vi "test-TimeInterpPose-Test1.vi"() -> (3 "All tests passed":bool)   [LabVIEW 2019]
uses:
  <vilib>/Rock Robotics/WPI/ThirdParty/JAS_Junk/TrajLib/POSE2D.ctl
  <vilib>/Rock Robotics/WPI/ThirdParty/JAS_Junk/TrajLib/TRANSLATION2D.ctl
  <vilib>/Rock Robotics/WPI/ThirdParty/JAS_Junk/TrajLib/ROTATION2D.ctl
  <vilib>/Rock Robotics/WPI/ThirdParty/JAS_Junk/TrajLib/Rotation2d_CreateAngle.vi
  <vilib>/Rock Robotics/WPI/ThirdParty/JAS_Junk/TrajLib/Translation2d_Create.vi
  <vilib>/Rock Robotics/WPI/ThirdParty/JAS_Junk/TrajLib/Translation2d_Equals.vi
  <vilib>/Rock Robotics/WPI/ThirdParty/JAS_Junk/TrajLib/Rotation2d_Equals.vi
  <vilib>/Rock Robotics/WPI/ThirdParty/JAS_Junk/TrajLib/TimeInterpPose2d_CleanUp.vi
  <vilib>/Rock Robotics/WPI/ThirdParty/JAS_Junk/TrajLib/Util_CalcDist.vi
  <vilib>/gmath/interp.llb/Search Ordered Table.vi
  <vilib>/Rock Robotics/WPI/ThirdParty/JAS_Junk/TrajLib/Trajectory_Library.lvlib
panel:
  out "out POSE 1.0":T1 {"ROTATION"."SIN" format="%13.4f"; "ROTATION"."COS" format="%13.4f"; "ROTATION"."VALUE" format="%13.4f"; "TRANSLATION"."Y" format="%14.3f"; "TRANSLATION"."X" format="%14.3f"}
  out "OutputPose 0.75":T1={"TRANSLATION"={"X"=0.0, "Y"=0.0}, "ROTATION"={"VALUE"=0.0, "COS"=1.0, "SIN"=0.0}} {"ROTATION"."SIN" format="%13.4f"; "ROTATION"."COS" format="%13.4f"; "ROTATION"."VALUE" format="%13.4f"; "TRANSLATION"."Y" format="%14.3f"; "TRANSLATION"."X" format="%14.3f"}
  out "out POSE  0.0":T1 {"ROTATION"."SIN" format="%13.4f"; "ROTATION"."COS" format="%13.4f"; "ROTATION"."VALUE" format="%13.4f"; "TRANSLATION"."Y" format="%14.3f"; "TRANSLATION"."X" format="%14.3f"}
  out "OutputPose 0.5":T1={"TRANSLATION"={"X"=0.0, "Y"=0.0}, "ROTATION"={"VALUE"=0.0, "COS"=1.0, "SIN"=0.0}} {"ROTATION"."SIN" format="%13.4f"; "ROTATION"."COS" format="%13.4f"; "ROTATION"."VALUE" format="%13.4f"; "TRANSLATION"."Y" format="%14.3f"; "TRANSLATION"."X" format="%14.3f"}
  out "OutputPose 0.25":T1={"TRANSLATION"={"X"=0.0, "Y"=0.0}, "ROTATION"={"VALUE"=0.0, "COS"=1.0, "SIN"=0.0}} {"ROTATION"."SIN" format="%13.4f"; "ROTATION"."COS" format="%13.4f"; "ROTATION"."VALUE" format="%13.4f"; "TRANSLATION"."Y" format="%14.3f"; "TRANSLATION"."X" format="%14.3f"}
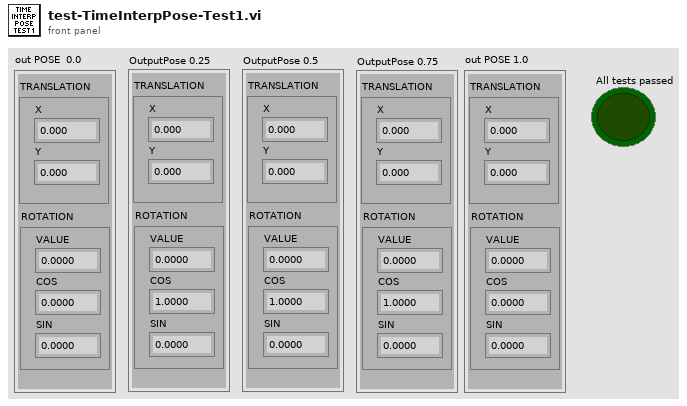
[diagram p1: front panel]
types:
  T1 = typedef "Trajectory_Library.lvlib/POSE2D.ctl" = cluster{"TRANSLATION":T2, "ROTATION":T3}
  T2 = typedef "Trajectory_Library.lvlib/TRANSLATION2D.ctl" = cluster{"X":dbl, "Y":dbl}
  T3 = typedef "Trajectory_Library.lvlib/ROTATION2D.ctl" = cluster{"VALUE":dbl, "COS":dbl, "SIN":dbl}
  T4 = typedef "Trajectory_Library.lvlib/TIME_INTERPOLATABLE_POSE.ctl" = cluster{"TimeStamps":dbl[], "Pose":T1[], "Min_TimeStamp":dbl, "Max_TimeStamp":dbl, "ItemCount":i32, "MaxBufferTime":dbl}
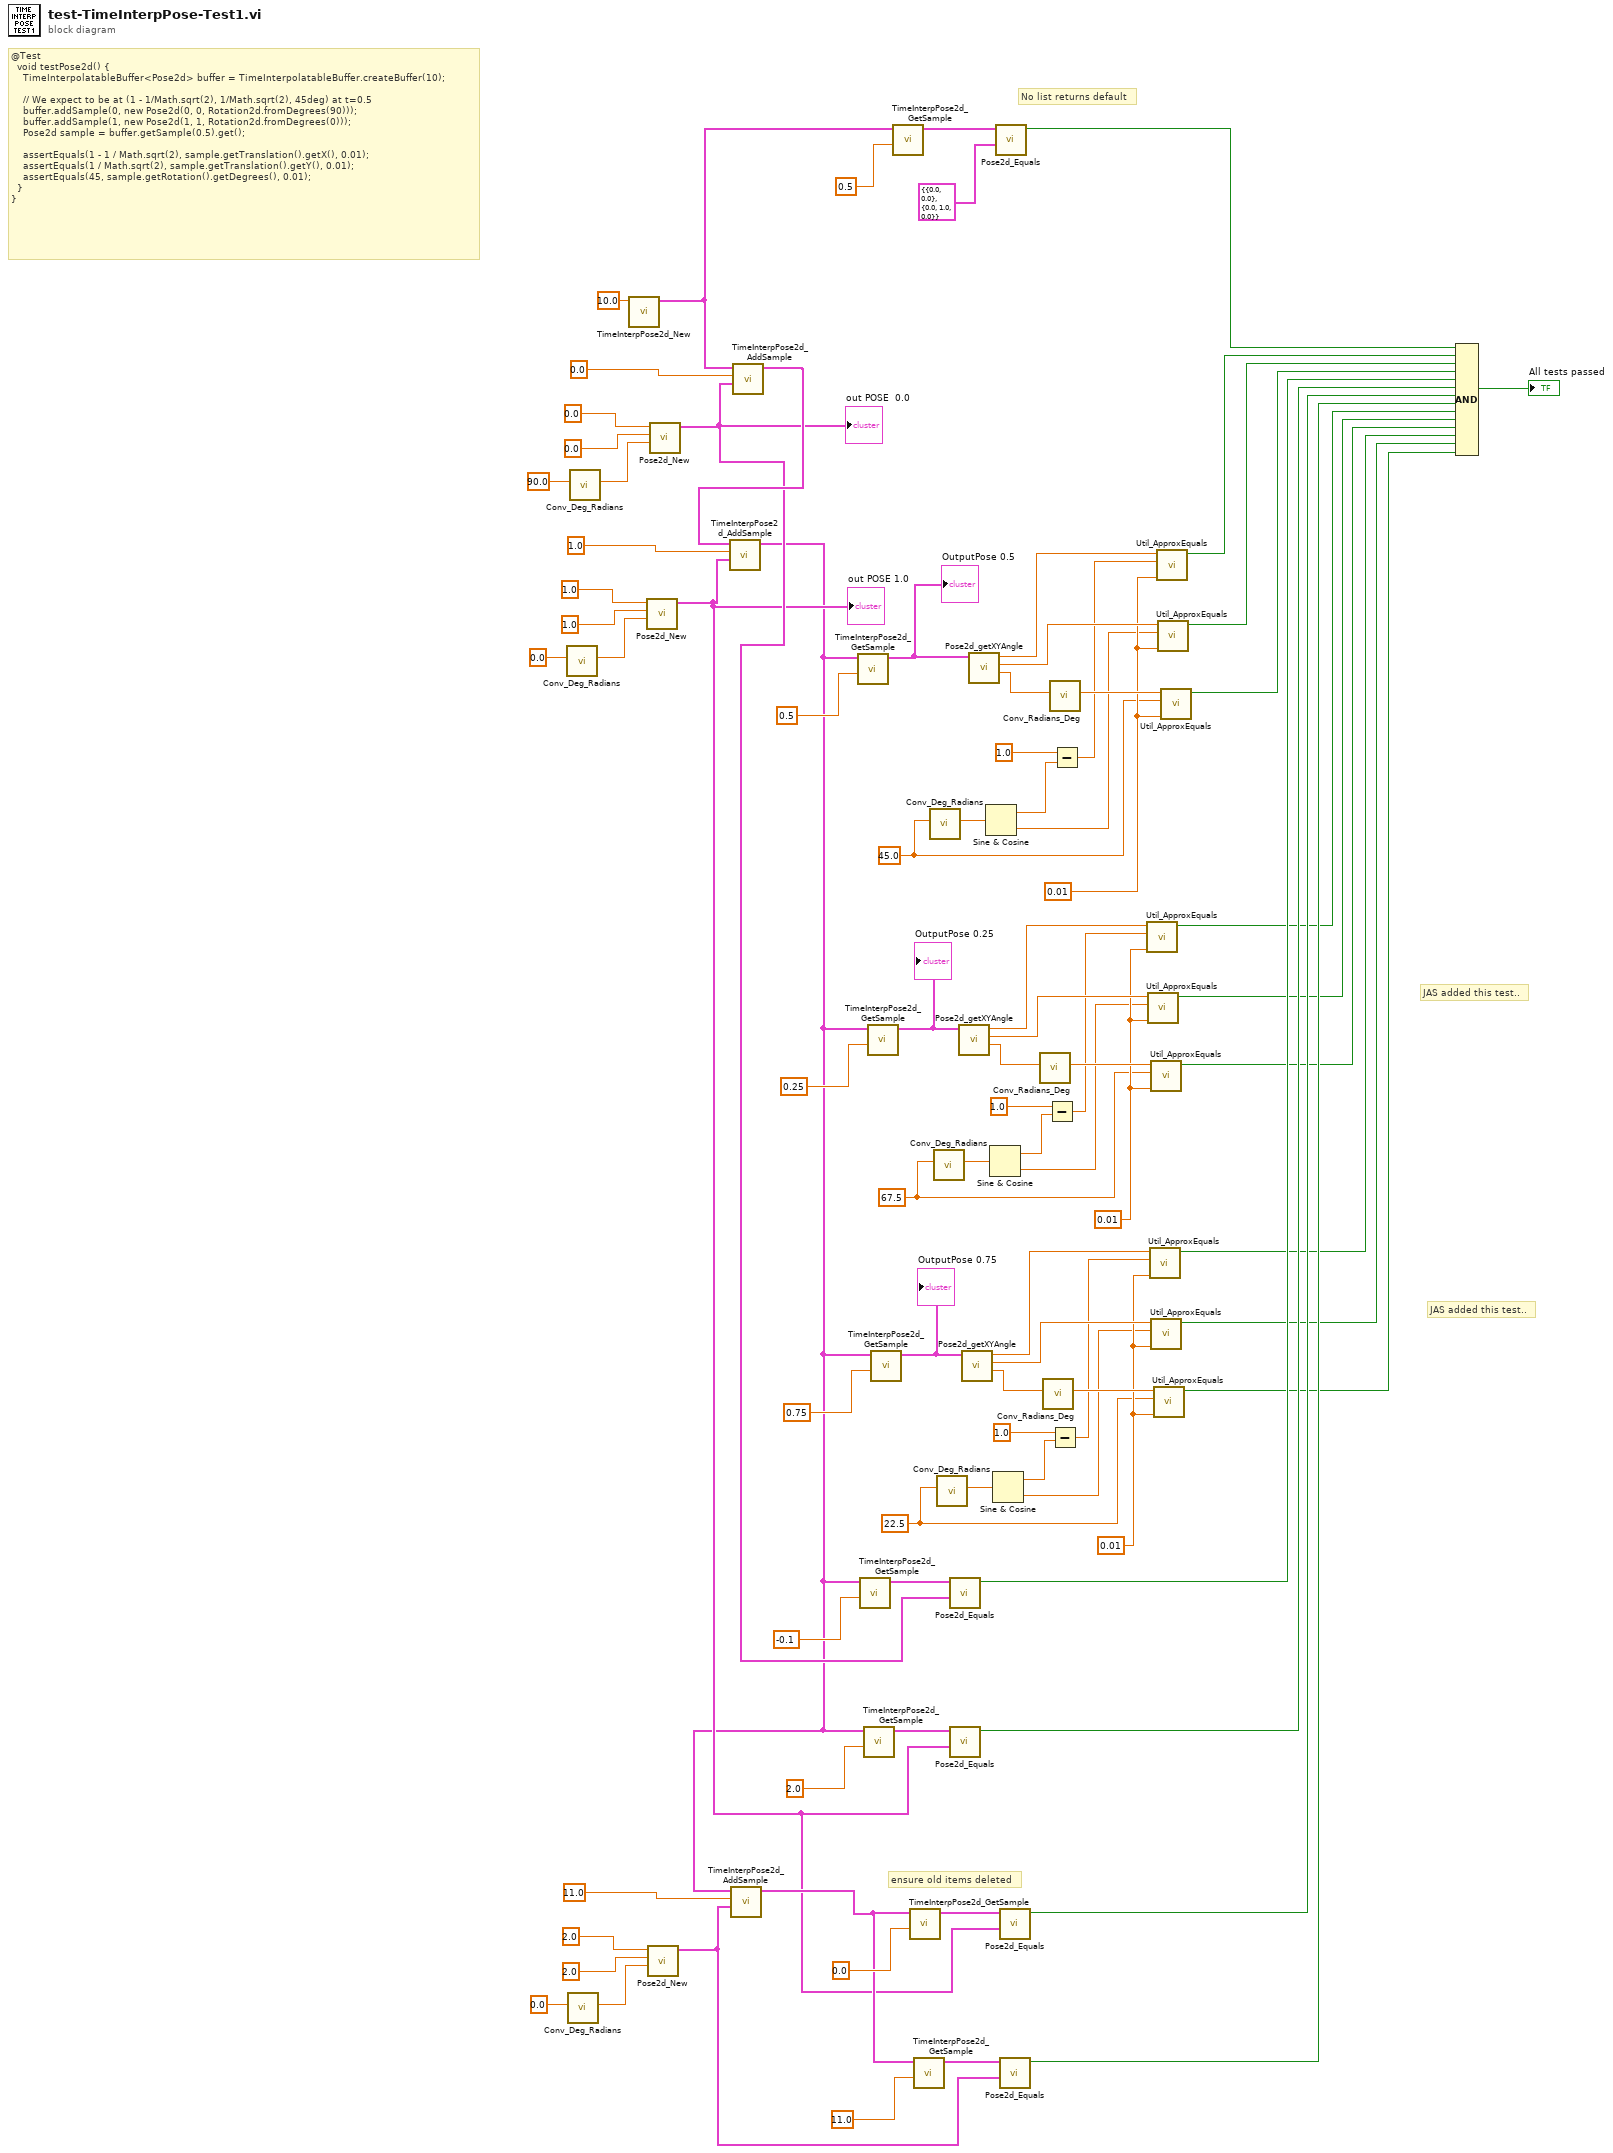
[diagram p0: block diagram]
diagram:
  w9 = 22.5 ("Value 2")
  w11 = 0.01 ("Tolerance")
  w24 = 67.5 ("Value 2")
  w31 = 0.01 ("Tolerance")
  w68 = 0.01 ("Tolerance")
  w27 = 45.0 ("Value 2")
  # "JAS added this test.."
  # "JAS added this test.."
  # "ensure old items deleted"
  # "No list returns default"
  # "@Test\n  void testPose2d() {\n    TimeInterpolatableBuffer<Pose2d> buffer = TimeInterpolatableBuffer.createBuffer(10);\n\n    // We expect to be at (1 - 1/Math.sqrt(2), 1/Math.sqrt(2), 45deg) at t=0.5\n    buffer.addSample(0, new Pose2d(0, 0, Rotation2d.fromDegrees(90)));\n    buffer.addSample(1, new Pose2d(1, 1, Rotation2d.fromDegrees(0)));\n    Pose2d sample = buffer.getSample(0.5).get();\n\n    assertEquals(1 - 1 / Math.sqrt(2), sample.getTranslation().getX(), 0.01);\n    assertEquals(1 / Math.sqrt(2), sample.getTranslation().getY(), 0.01);\n    assertEquals(45, sample.getRotation().getDegrees(), 0.01);\n  }\n}"
  n1 = call <vilib>:"Conv_Deg_Radians.vi"("Degress"=0.0) -> ("Radians"=w79:dbl)  [unwired: 10 in]
  n2 = call <vilib>:"Conv_Deg_Radians.vi"("Degress"=0.0) -> ("Radians"=w49:dbl)  [unwired: 10 in]
  n3 = call <vilib>:"Conv_Deg_Radians.vi"("Degress"=90.0) -> ("Radians"=w84:dbl)  [unwired: 10 in]
  n4 = call <vilib>:"TimeInterpPose2d_New.vi"("MaxTime"=10.0) -> ("TimeInterpPose"=w60:T4)  [unwired: 10 in]
  n5 = call <vilib>:"Pose2d_New.vi"("Heading"=w79, "Y"=1.0, "X"=1.0) -> ("out POSe"=w38:T1)  [unwired: 8 in]
  "out POSE 1.0" <- w38
  n6 = call <vilib>:"Pose2d_New.vi"("Heading"=w49, "Y"=2.0, "X"=2.0) -> ("out POSe"=w41:T1)  [unwired: 8 in]
  n7 = call <vilib>:"Pose2d_New.vi"("Heading"=w84, "Y"=0.0, "X"=0.0) -> ("out POSe"=w56:T1)  [unwired: 8 in]
  "out POSE  0.0" <- w56
  n8 = call <vilib>:"TimeInterpPose2d_AddSample.vi"("Pose"=w56, "TimeStamp"=0.0, "in TimeInterpPose"=w60) -> ("out TimeInterpPose"=w63:T4)  [unwired: 7 in, 1 out]
  n9 = call <vilib>:"TimeInterpPose2d_AddSample.vi"("Pose"=w38, "TimeStamp"=1.0, "in TimeInterpPose"=w63) -> ("out TimeInterpPose"=w4:T4)  [unwired: 7 in, 1 out]
  n10 = call <vilib>:"TimeInterpPose2d_AddSample.vi"("Pose"=w41, "TimeStamp"=11.0, "in TimeInterpPose"=w4) -> ("out TimeInterpPose"=w42:T4)  [unwired: 7 in, 1 out]
  n11 = call <vilib>:"TimeInterpPose2d_GetSample.vi"("TimeStamp"=0.5, "TimeInterpPose"=w4) -> ("OutputPose"=w75:T1)  [unwired: 9 in]
  "OutputPose 0.5" <- w75
  n12 = call <vilib>:"TimeInterpPose2d_GetSample.vi"("TimeStamp"=-0.1, "TimeInterpPose"=w4) -> ("OutputPose"=w57:T1)  [unwired: 9 in]
  n13 = call <vilib>:"TimeInterpPose2d_GetSample.vi"("TimeStamp"=2.0, "TimeInterpPose"=w4) -> ("OutputPose"=w54:T1)  [unwired: 9 in]
  n14 = call <vilib>:"TimeInterpPose2d_GetSample.vi"("TimeStamp"=0.25, "TimeInterpPose"=w4) -> ("OutputPose"=w32:T1)  [unwired: 9 in]
  "OutputPose 0.25" <- w32
  n15 = call <vilib>:"TimeInterpPose2d_GetSample.vi"("TimeStamp"=0.75, "TimeInterpPose"=w4) -> ("OutputPose"=w12:T1)  [unwired: 9 in]
  "OutputPose 0.75" <- w12
  n16 = call <vilib>:"TimeInterpPose2d_GetSample.vi"("TimeStamp"=0.5, "TimeInterpPose"=w60) -> ("OutputPose"=w62:T1)  [unwired: 9 in]
  n17 = call <vilib>:"TimeInterpPose2d_GetSample.vi"("TimeStamp"=0.0, "TimeInterpPose"=w42) -> ("OutputPose"=w45:T1)  [unwired: 9 in]
  n18 = call <vilib>:"TimeInterpPose2d_GetSample.vi"("TimeStamp"=11.0, "TimeInterpPose"=w42) -> ("OutputPose"=w43:T1)  [unwired: 9 in]
  n19 = call <vilib>:"Conv_Deg_Radians.vi"("Degress"=w27) -> ("Radians"=w26:dbl)  [unwired: 10 in]
  n20 = call <vilib>:"Conv_Deg_Radians.vi"("Degress"=w24) -> ("Radians"=w25:dbl)  [unwired: 10 in]
  n21 = call <vilib>:"Conv_Deg_Radians.vi"("Degress"=w9) -> ("Radians"=w10:dbl)  [unwired: 10 in]
  n22 = call <vilib>:"Pose2d_Equals.vi"("other POSE"=w56, "in POSE"=w57) -> ("Equals"=w53:bool)  [unwired: 9 in]
  n23 = call <vilib>:"Pose2d_Equals.vi"("other POSE"=w38, "in POSE"=w54) -> ("Equals"=w52:bool)  [unwired: 9 in]
  n24 = call <vilib>:"Pose2d_getXYAngle.vi"("in POSE"=w32) -> ("Angle"=w36:dbl, "Y"=w34:dbl, "X"=w33:dbl)  [unwired: 8 in]
  n25 = call <vilib>:"Pose2d_getXYAngle.vi"("in POSE"=w12) -> ("Angle"=w16:dbl, "Y"=w14:dbl, "X"=w13:dbl)  [unwired: 8 in]
  n26 = call <vilib>:"Pose2d_getXYAngle.vi"("in POSE"=w75) -> ("Angle"=w74:dbl, "Y"=w72:dbl, "X"=w71:dbl)  [unwired: 8 in]
  n27 = Sine & Cosine(0:w26) -> (1:w19:dbl, 2:w18:dbl)
  n28 = Sine & Cosine(0:w25) -> (1:w21:dbl, 2:w20:dbl)
  n29 = Sine & Cosine(0:w10) -> (1:w6:dbl, 2:w5:dbl)
  n30 = call <vilib>:"Pose2d_Equals.vi"("other POSE"=T1 {"TRANSLATION"={"X"=0.0, "Y"=0.0}, "ROTATION"={"VALUE"=0.0, "COS"=1.0, "SIN"=0.0}} ("POSE"), "in POSE"=w62) -> ("Equals"=w61:bool)  [unwired: 9 in]
  n31 = call <vilib>:"Pose2d_Equals.vi"("other POSE"=w38, "in POSE"=w45) -> ("Equals"=w40:bool)  [unwired: 9 in]
  n32 = call <vilib>:"Pose2d_Equals.vi"("other POSE"=w41, "in POSE"=w43) -> ("Equals"=w39:bool)  [unwired: 9 in]
  n33 = call <vilib>:"Conv_Radians_Deg.vi"("Radians"=w36) -> ("Degrees"=w35:dbl)  [unwired: 10 in]
  n34 = call <vilib>:"Conv_Radians_Deg.vi"("Radians"=w16) -> ("Degrees"=w15:dbl)  [unwired: 10 in]
  n35 = Subtract(x=1.0, y=w21) -> (x-y=w22:dbl)
  n36 = call <vilib>:"Conv_Radians_Deg.vi"("Radians"=w74) -> ("Degrees"=w73:dbl)  [unwired: 10 in]
  n37 = Subtract(x=1.0, y=w6) -> (x-y=w7:dbl)
  n38 = Subtract(x=1.0, y=w19) -> (x-y=w69:dbl)
  n39 = call <vilib>:"Util_ApproxEquals.vi"("Tolerance"=w31, "Value 2"=w22, "Value 1"=w33) -> ("ApproxEquals"=w30:bool)  [unwired: 8 in]
  n40 = call <vilib>:"Util_ApproxEquals.vi"("Tolerance"=w31, "Value 2"=w20, "Value 1"=w34) -> ("ApproxEquals"=w29:bool)  [unwired: 8 in]
  n41 = call <vilib>:"Util_ApproxEquals.vi"("Tolerance"=w11, "Value 2"=w7, "Value 1"=w13) -> ("ApproxEquals"=w3:bool)  [unwired: 8 in]
  n42 = call <vilib>:"Util_ApproxEquals.vi"("Tolerance"=w31, "Value 2"=w24, "Value 1"=w35) -> ("ApproxEquals"=w28:bool)  [unwired: 8 in]
  n43 = call <vilib>:"Util_ApproxEquals.vi"("Tolerance"=w11, "Value 2"=w5, "Value 1"=w14) -> ("ApproxEquals"=w2:bool)  [unwired: 8 in]
  n44 = call <vilib>:"Util_ApproxEquals.vi"("Tolerance"=w11, "Value 2"=w9, "Value 1"=w15) -> ("ApproxEquals"=w1:bool)  [unwired: 8 in]
  n45 = call <vilib>:"Util_ApproxEquals.vi"("Tolerance"=w68, "Value 2"=w69, "Value 1"=w71) -> ("ApproxEquals"=w67:bool)  [unwired: 8 in]
  n46 = call <vilib>:"Util_ApproxEquals.vi"("Tolerance"=w68, "Value 2"=w18, "Value 1"=w72) -> ("ApproxEquals"=w66:bool)  [unwired: 8 in]
  n47 = call <vilib>:"Util_ApproxEquals.vi"("Tolerance"=w68, "Value 2"=w27, "Value 1"=w73) -> ("ApproxEquals"=w65:bool)  [unwired: 8 in]
  n48 = Compound Arithmetic op=AND(w61, w67, w66, w65, w53, w52, w40, w39, w30, w29, w28, w3, w2, w1) -> (→"All tests passed":bool)
